vi "IQA check.vi"(8 "CHANGE":refnum<user-event>, 11 "connection in":T1) -> (3 "connection out":T1)   [LabVIEW 2017]
uses:
  <vilib>/addons/database/Connection.llb/Conn ObjectReference.ctl
  Control/State machine.ctl
  <vilib>/Utility/miscctls.llb/LVPointTypeDef.ctl
  <vilib>/addons/database/Connection.llb/Conn Execute.vi
  <vilib>/addons/database/Recordset.llb/Rec Fetch Recordset Data (R).vi
  <vilib>/addons/database/Recordset.llb/Rec Destroy - Connection.vi
  <vilib>/addons/database/_DB Variant To Data/Database Variant To Data.xnode
  <vilib>/addons/database/NI_Database_API.lvlib
  <vilib>/addons/database/Connection.llb/DB Tools Open Connec (Path).vi
panel:
  out "stock":string
  out "Ex-Im Code":string
  out "offset":string
  in  "Tab Control":enum32{"Main", "Debug"}(tab)
  in  "Level of shipment":string(combo)="N"
  in  "NG":bool
  in  "OK":bool
  out "Result":bool
  in  "Maker Code 2":string caption="Maker Code"
  out "Item Code 2":string caption="Item Code"
  in  "Barcode (F2)":string
  out "Maker Code":string
  out "Item Code":string
  in  "QR-Code (F1)":string
  out "ECODE":string
  # "IQA CHECK"
  # "QUALITY"
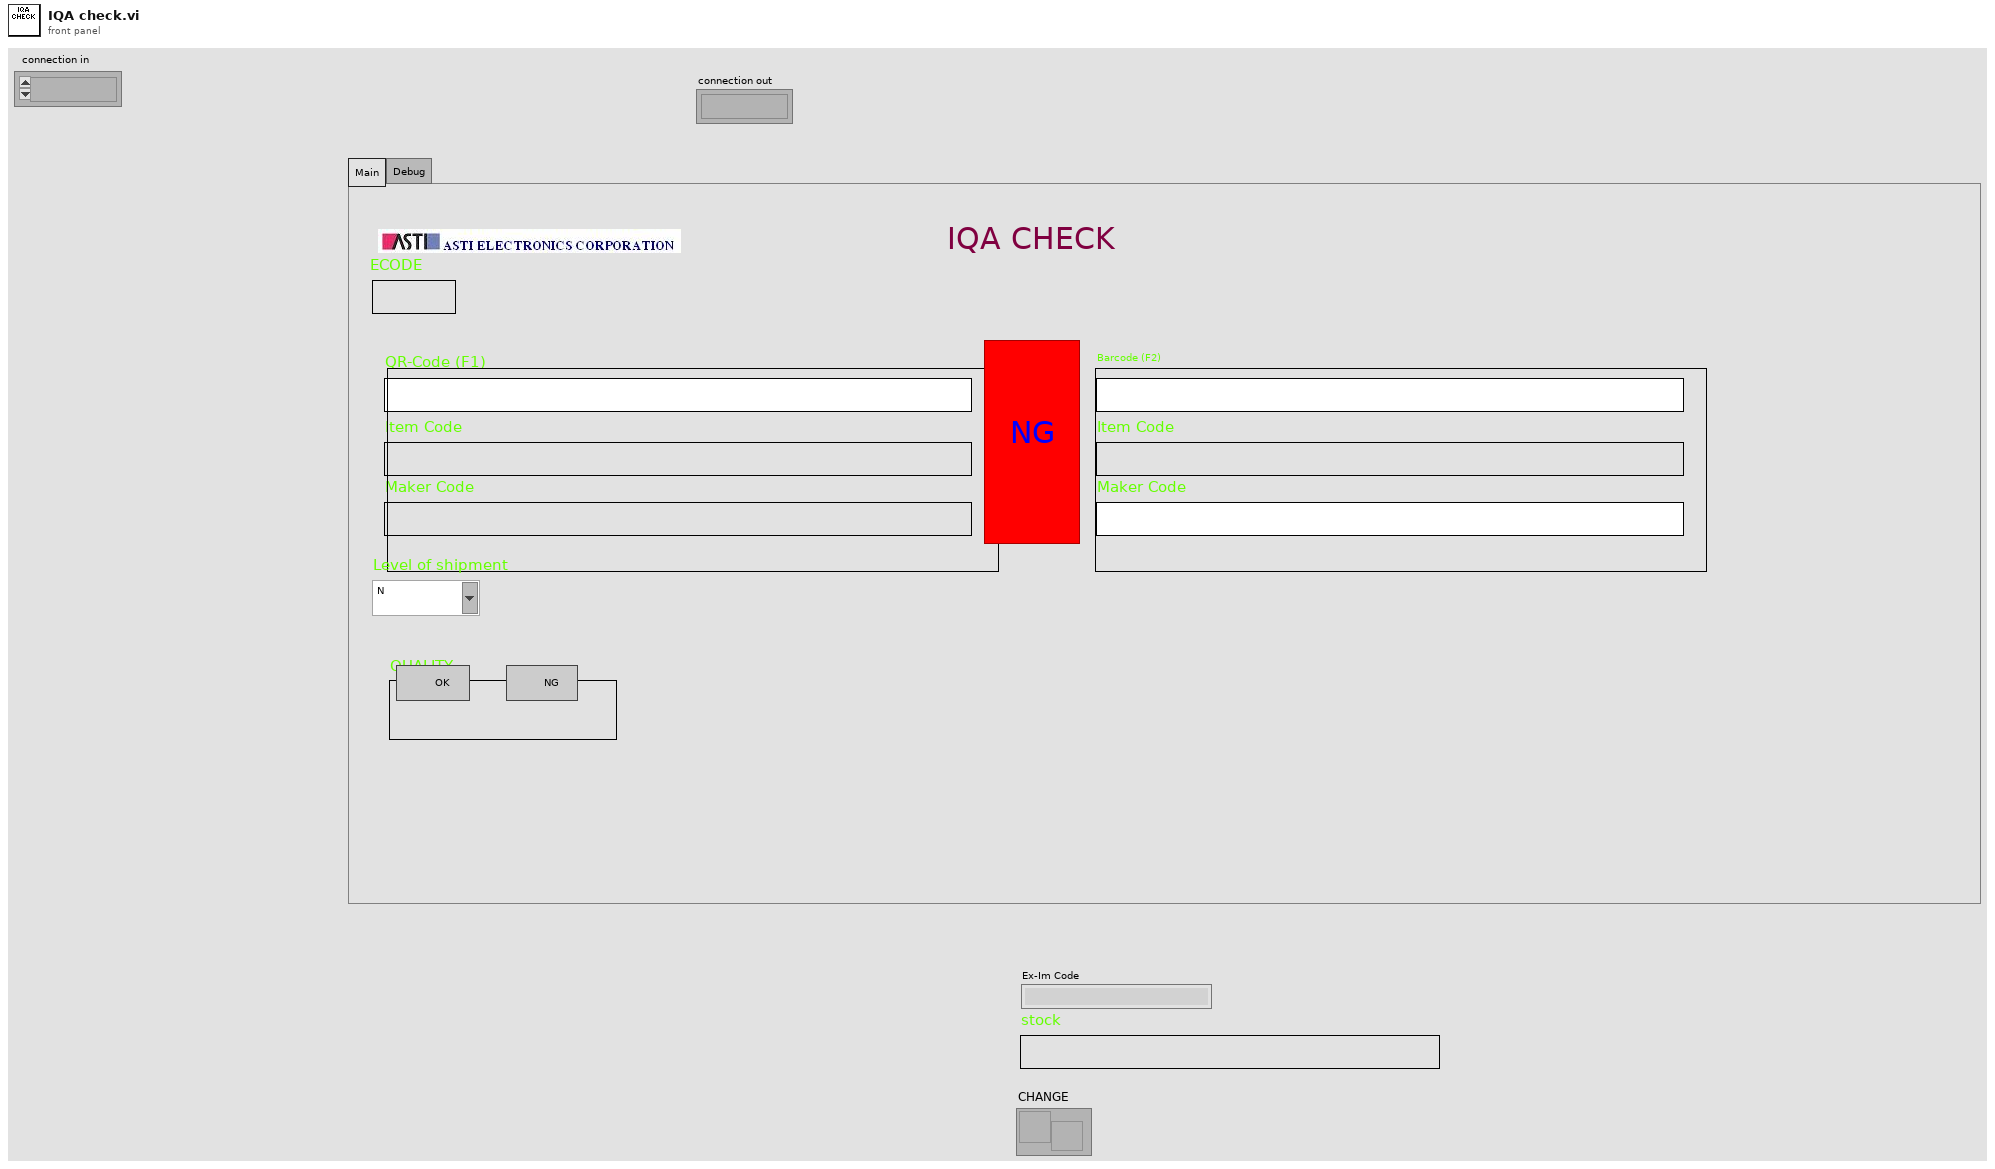
[diagram p1: front panel]
types:
  T1 = typedef "NI_Database_API.lvlib/Conn ObjectReference.ctl" = refnum<k1>
  T2 = enum8{"Enabled", "Disabled", "Disabled and Grayed Out"}
  T3 = typedef "LVPointTypeDef.ctl" = cluster{"Horizontal":i16, "Vertical":i16}
  T4 = typedef "State machine.ctl" = enum16{"Licence check", "Initial", "Log in", "Creat Config file", "Network setting", "Creat database 1", "Creat database 2", "Creat database 3", "Transfer", "Begin", "Exit"}
  T5 = typedef "NI_Database_API.lvlib/Rec ObjectReference.ctl" = refnum<k1>
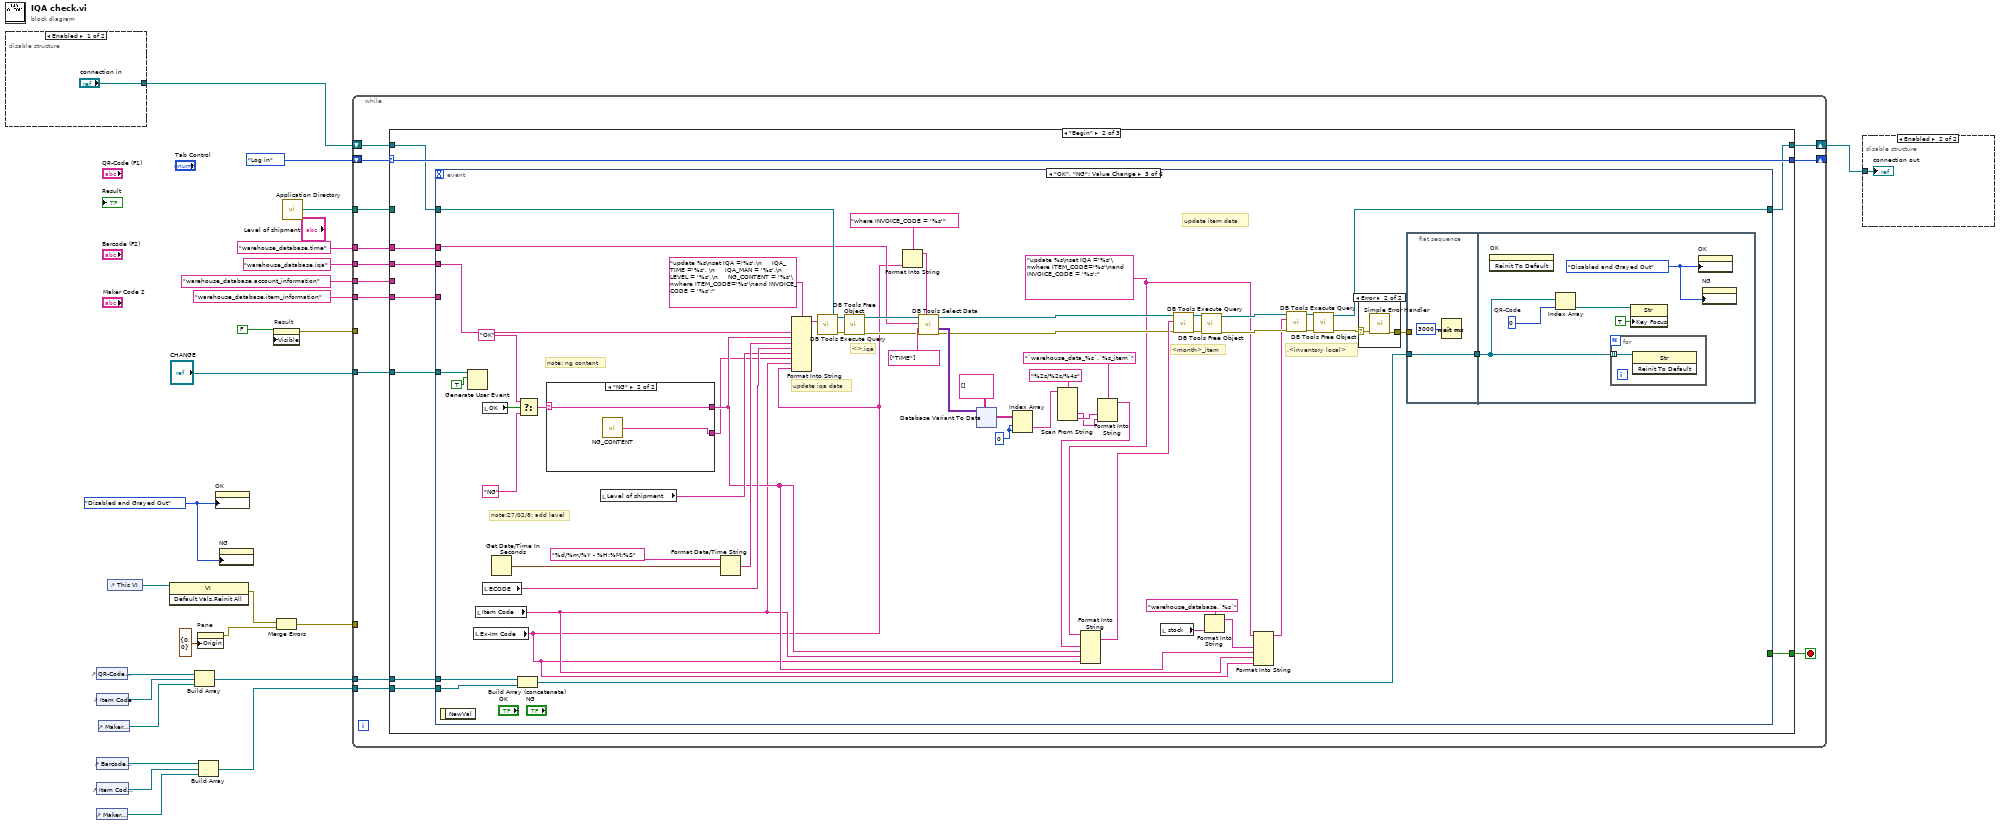
[diagram p0: block diagram]
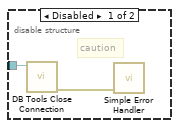
[diagram p2: hidden frame]
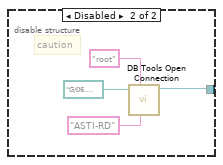
[diagram p3: hidden frame]
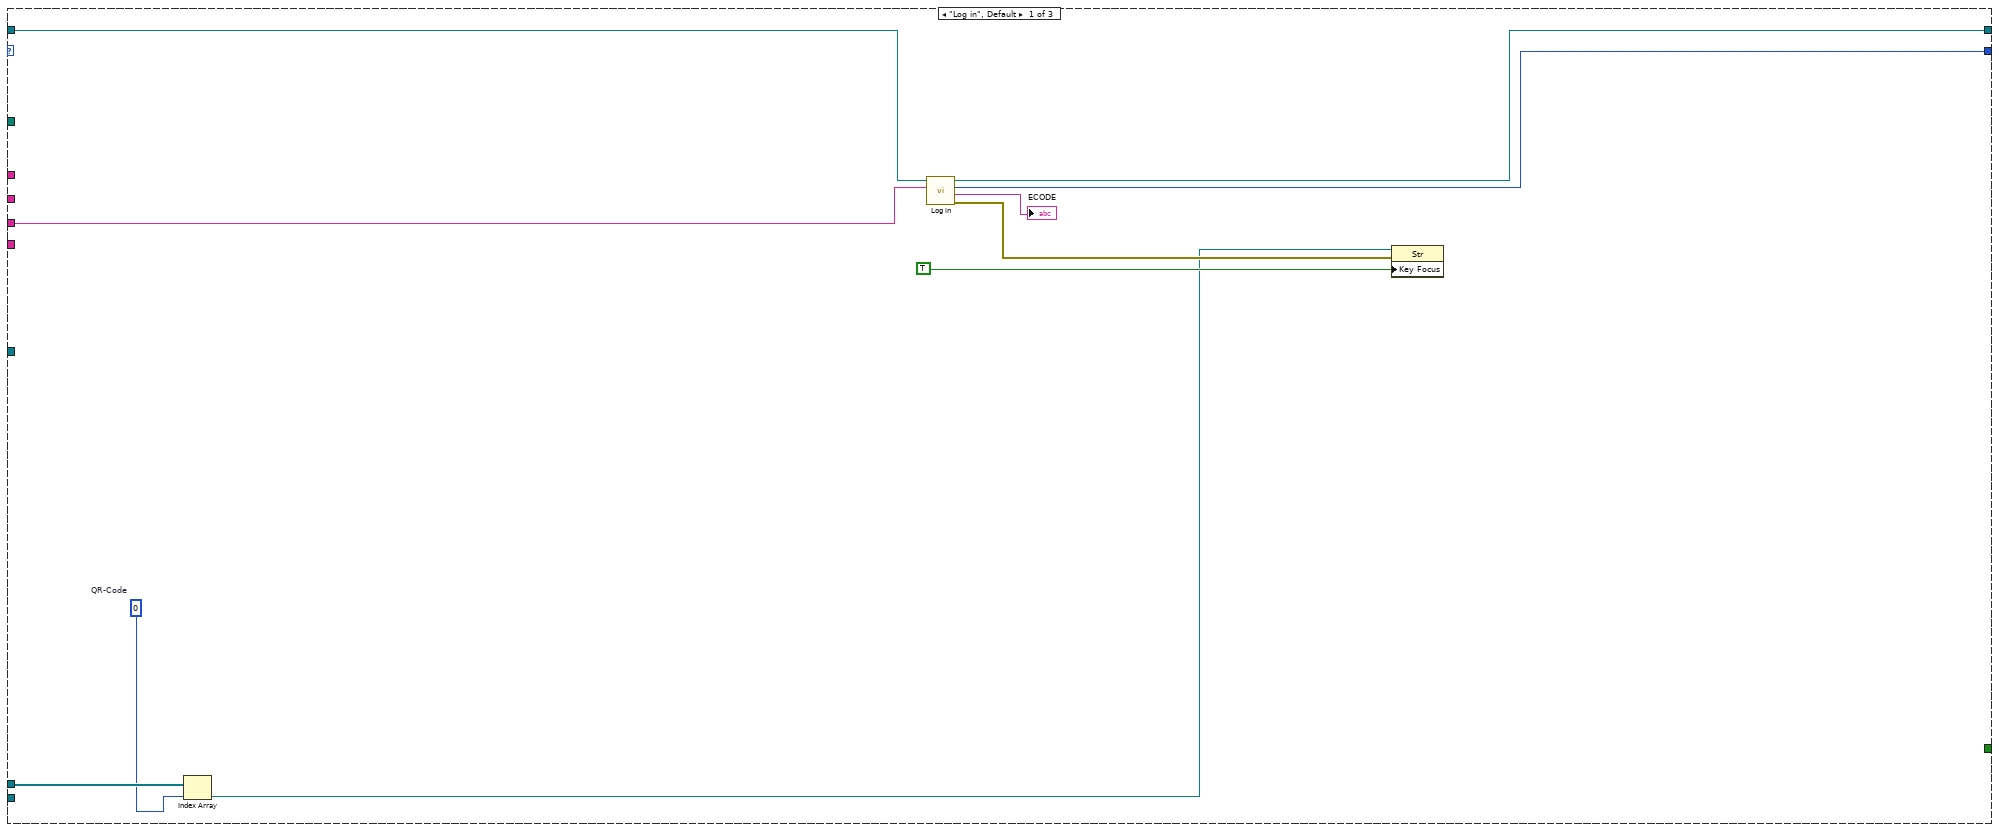
[diagram p4: hidden frame]
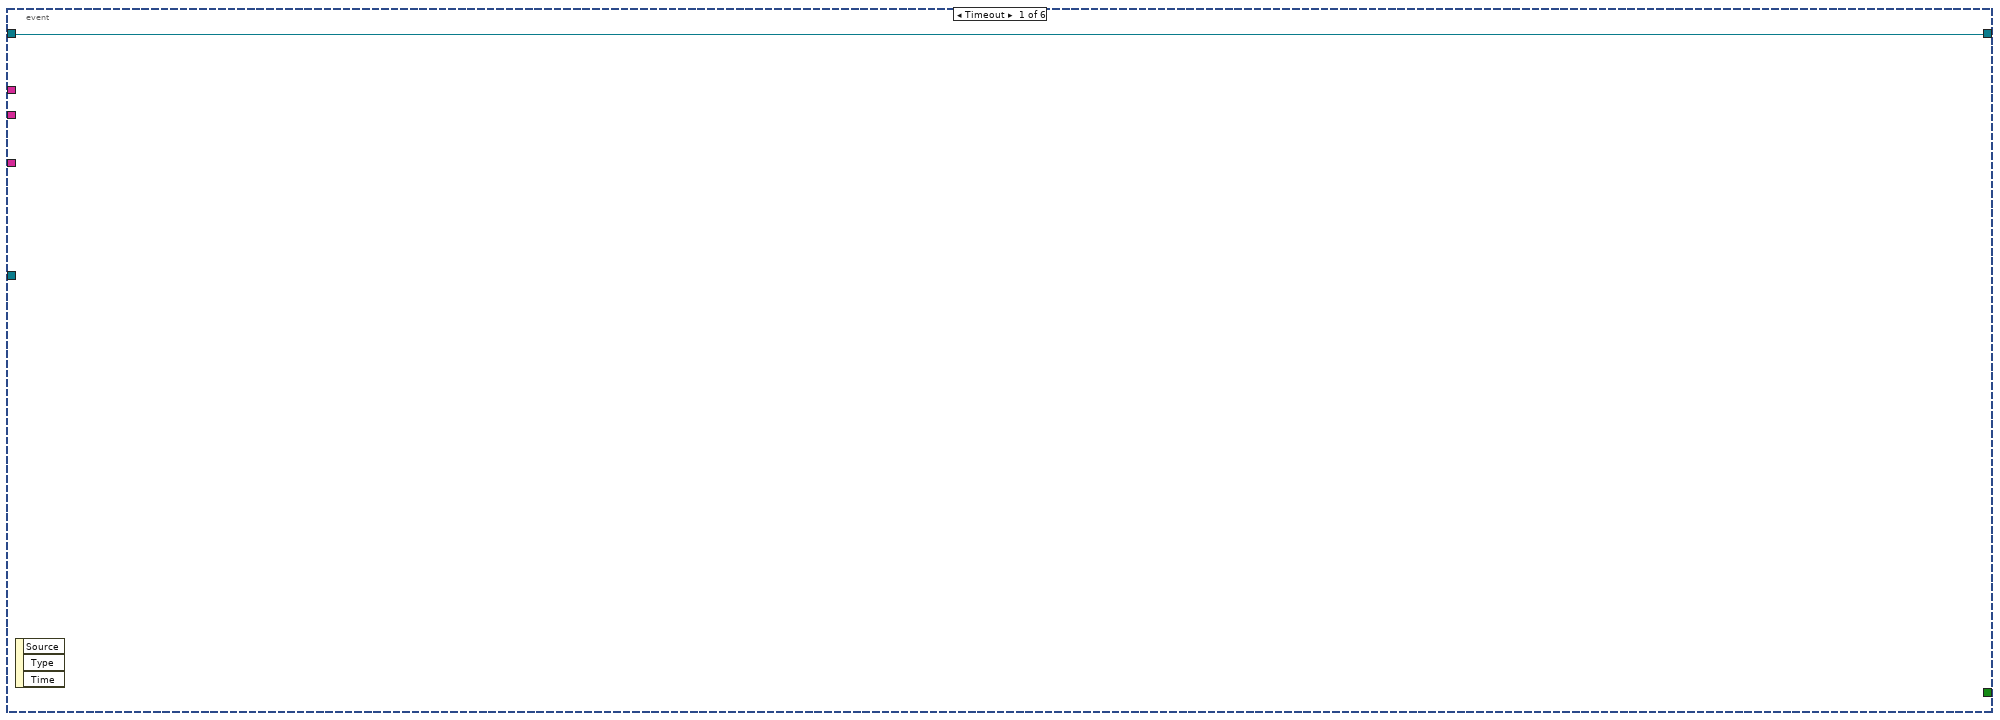
[diagram p5: hidden frame]
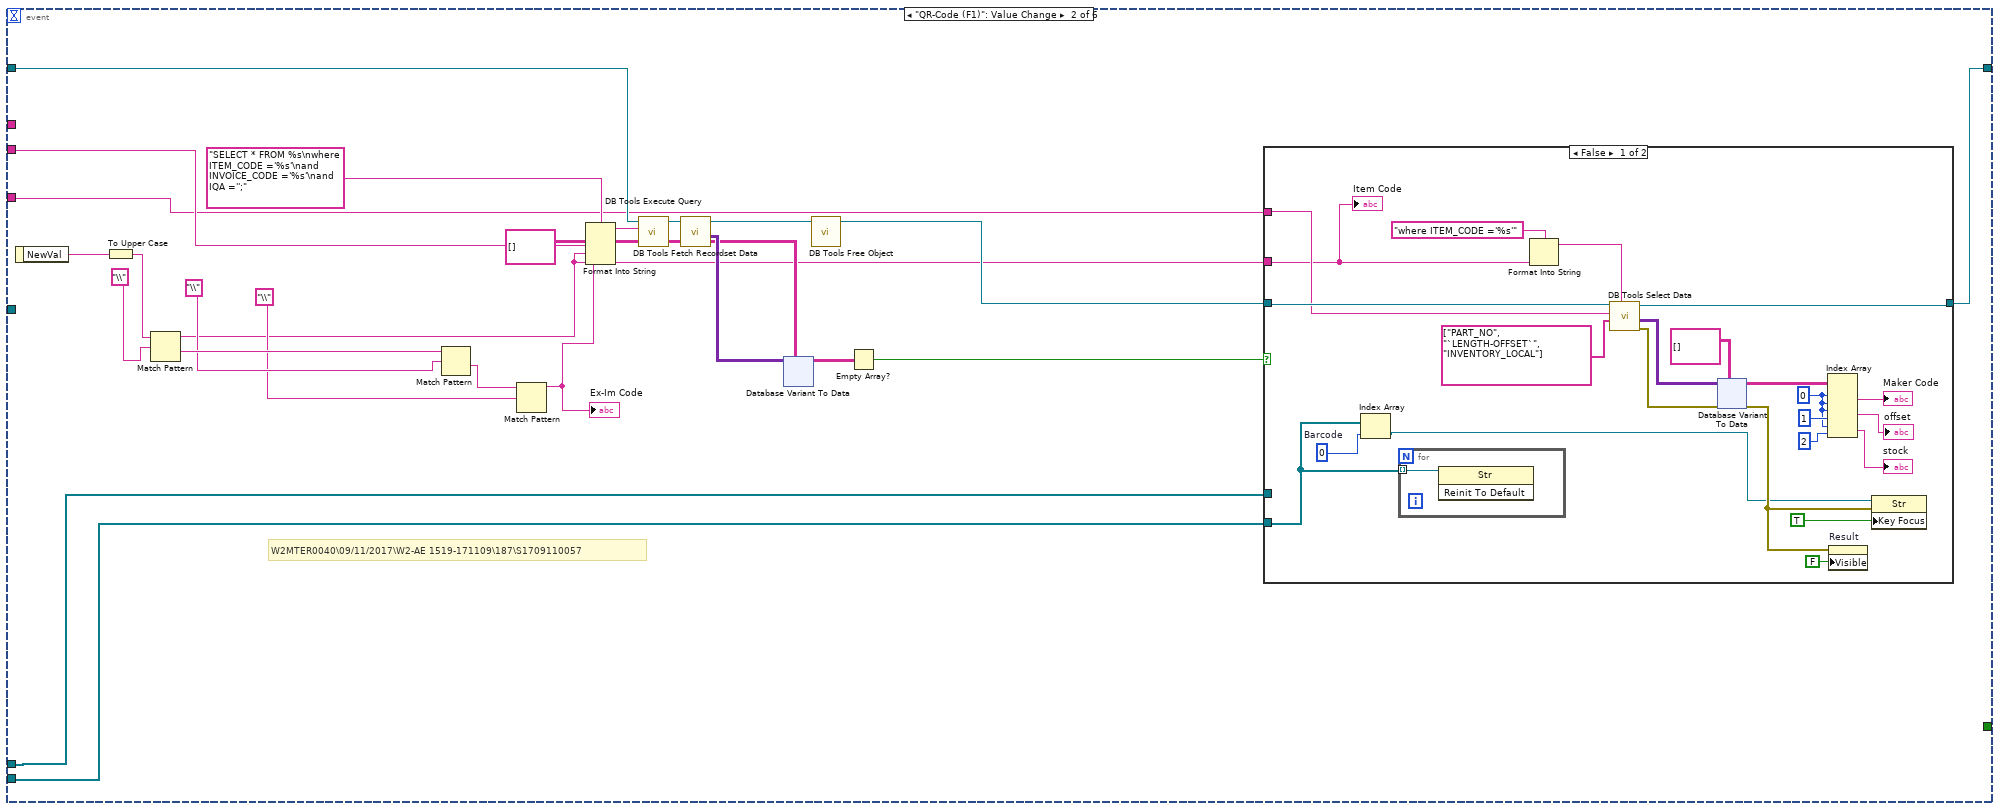
[diagram p6: hidden frame]
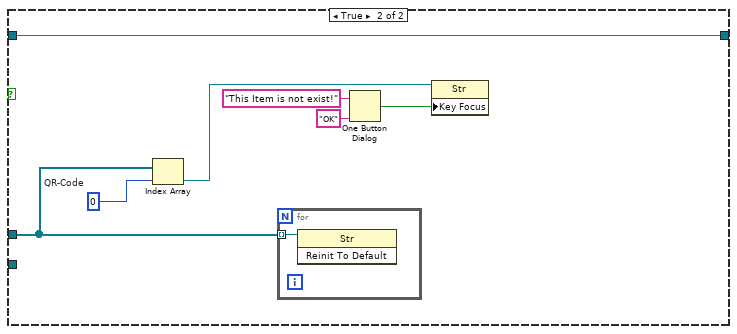
[diagram p7: hidden frame]
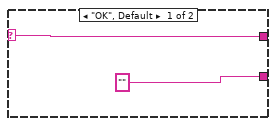
[diagram p8: hidden frame]
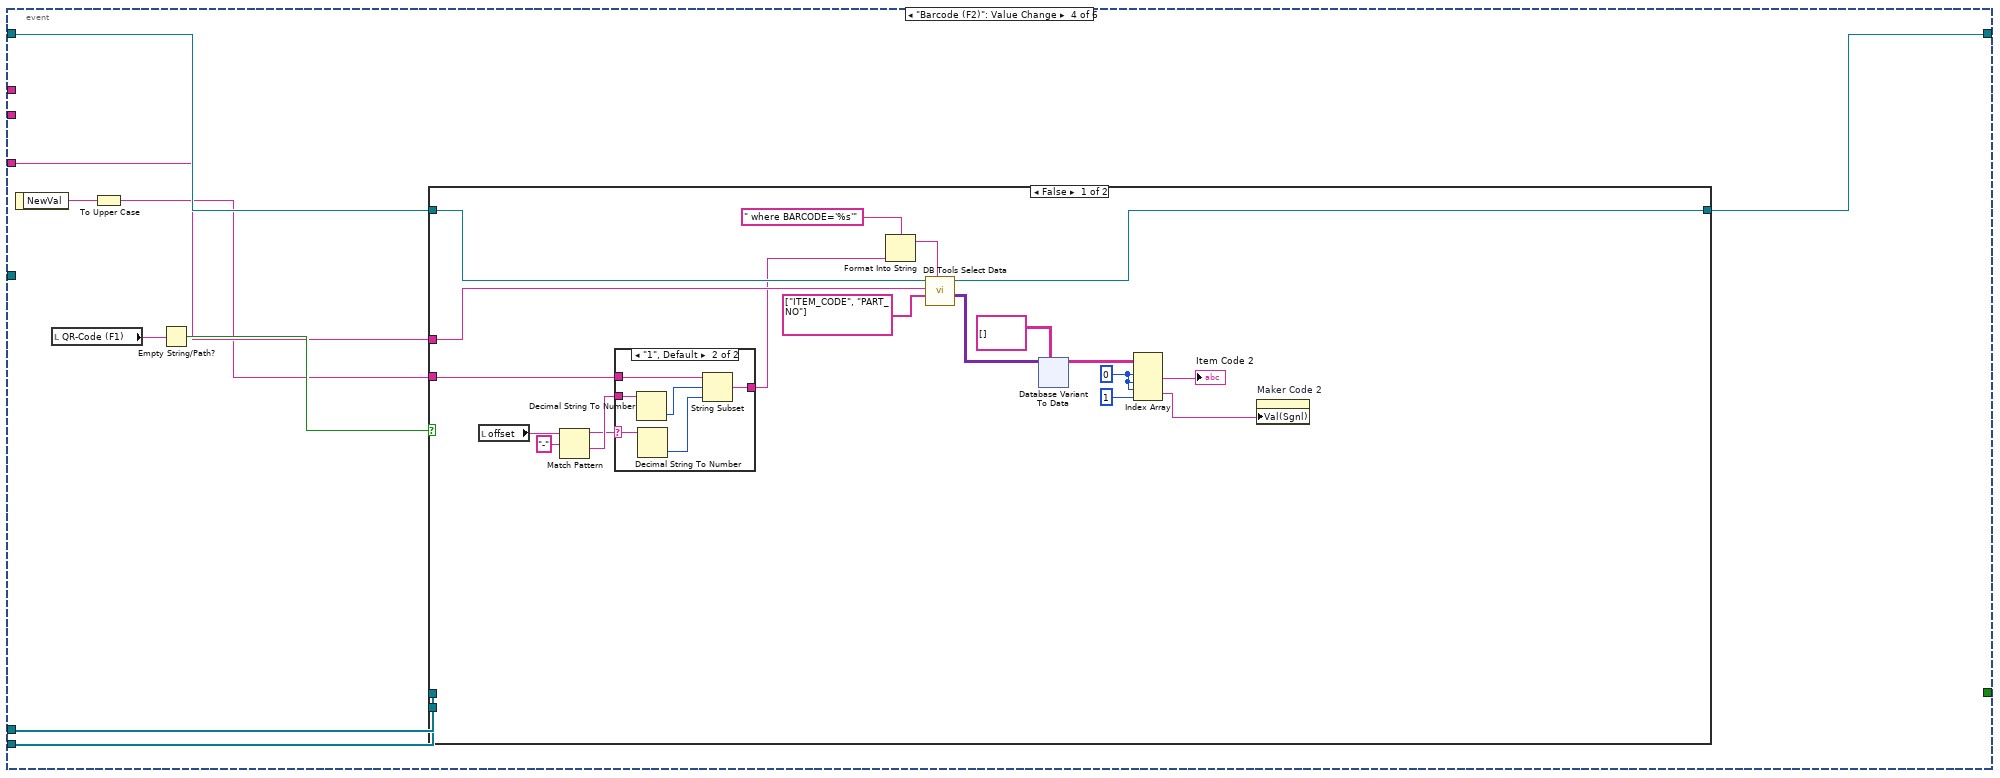
[diagram p10: hidden frame]
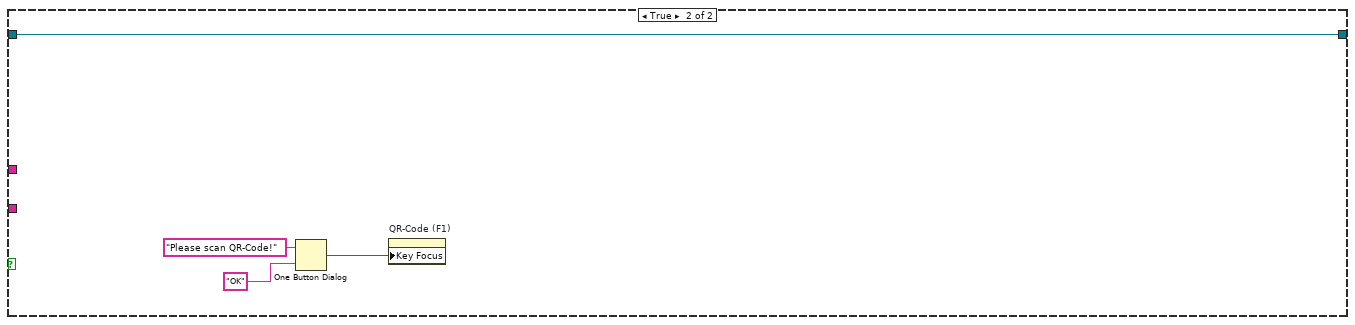
[diagram p12: hidden frame]
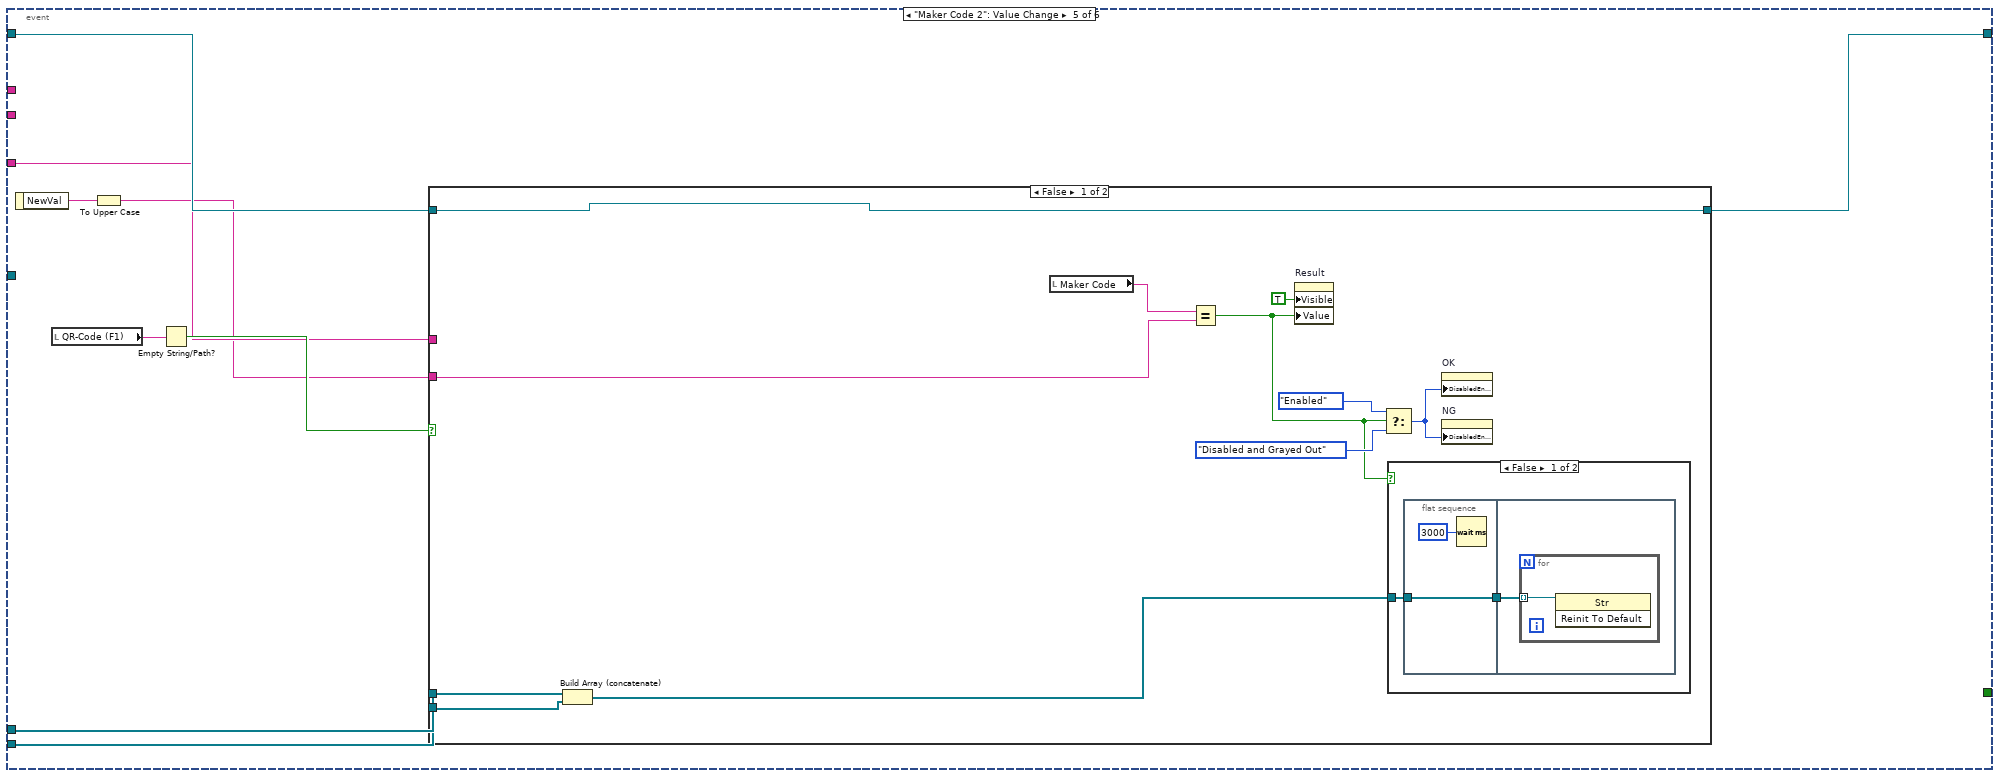
[diagram p13: hidden frame]
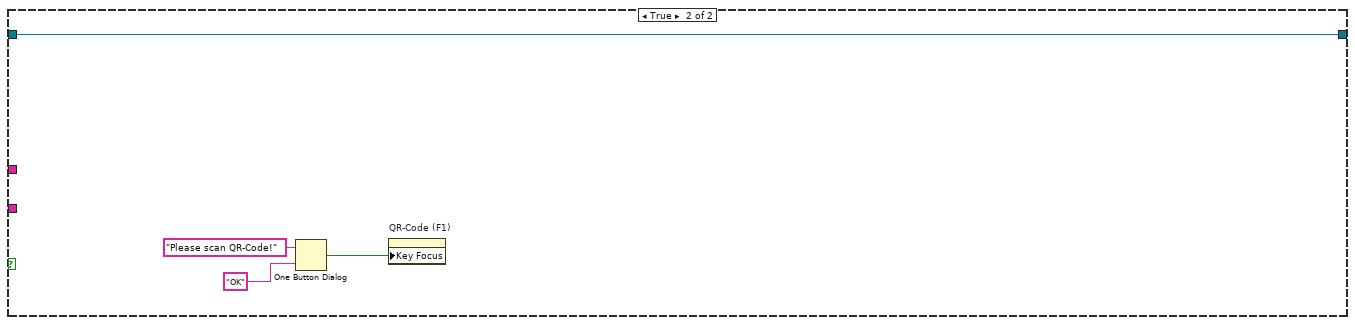
[diagram p15: hidden frame]
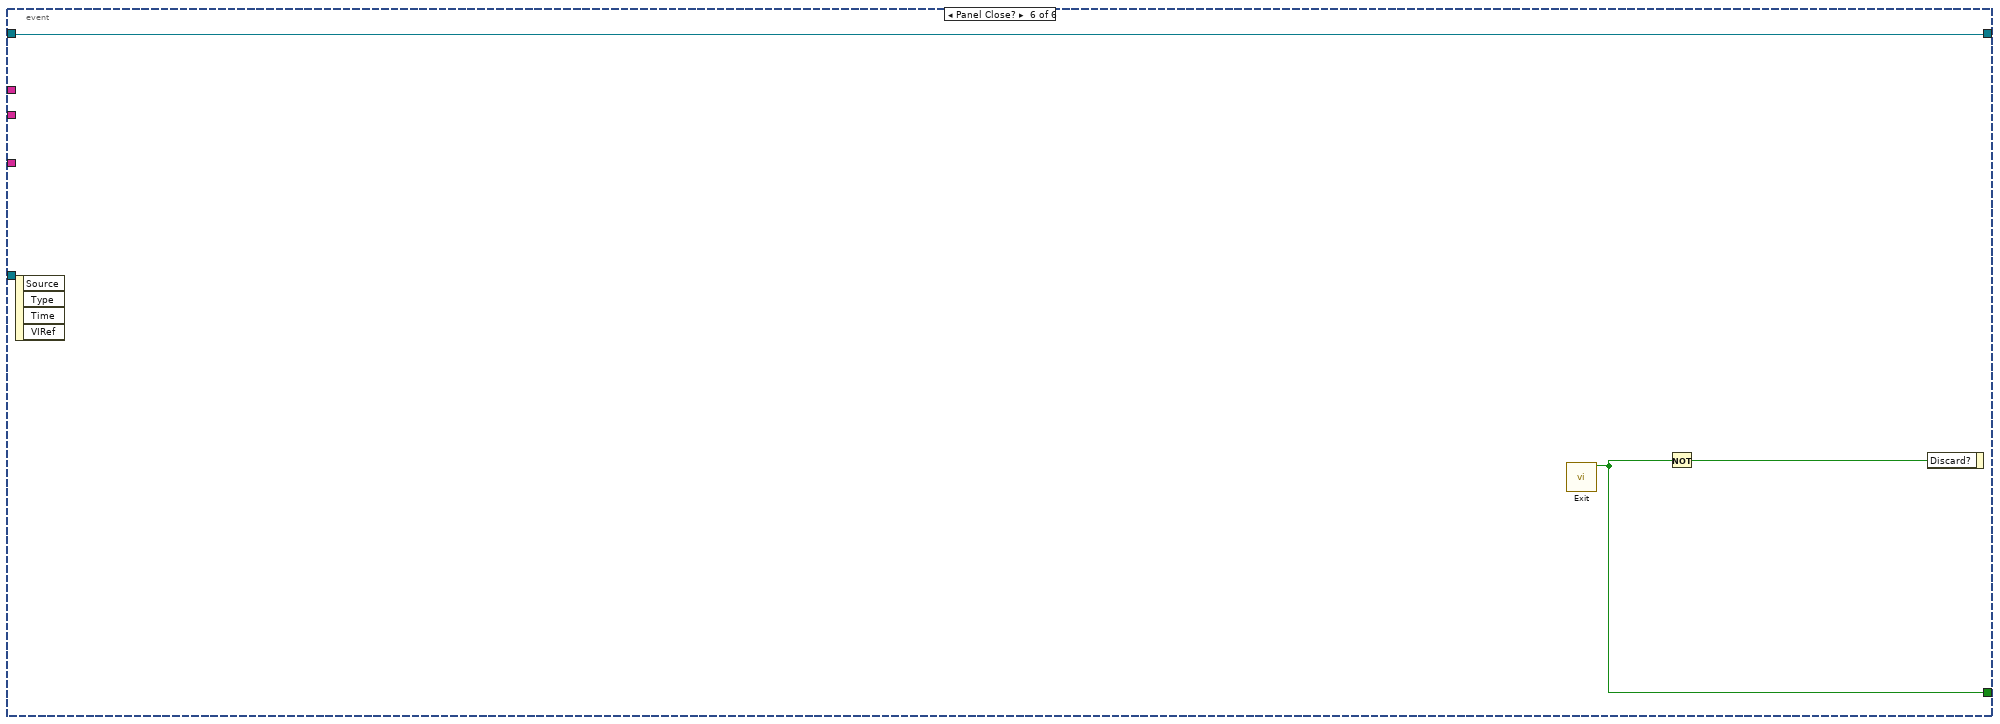
[diagram p16: hidden frame]
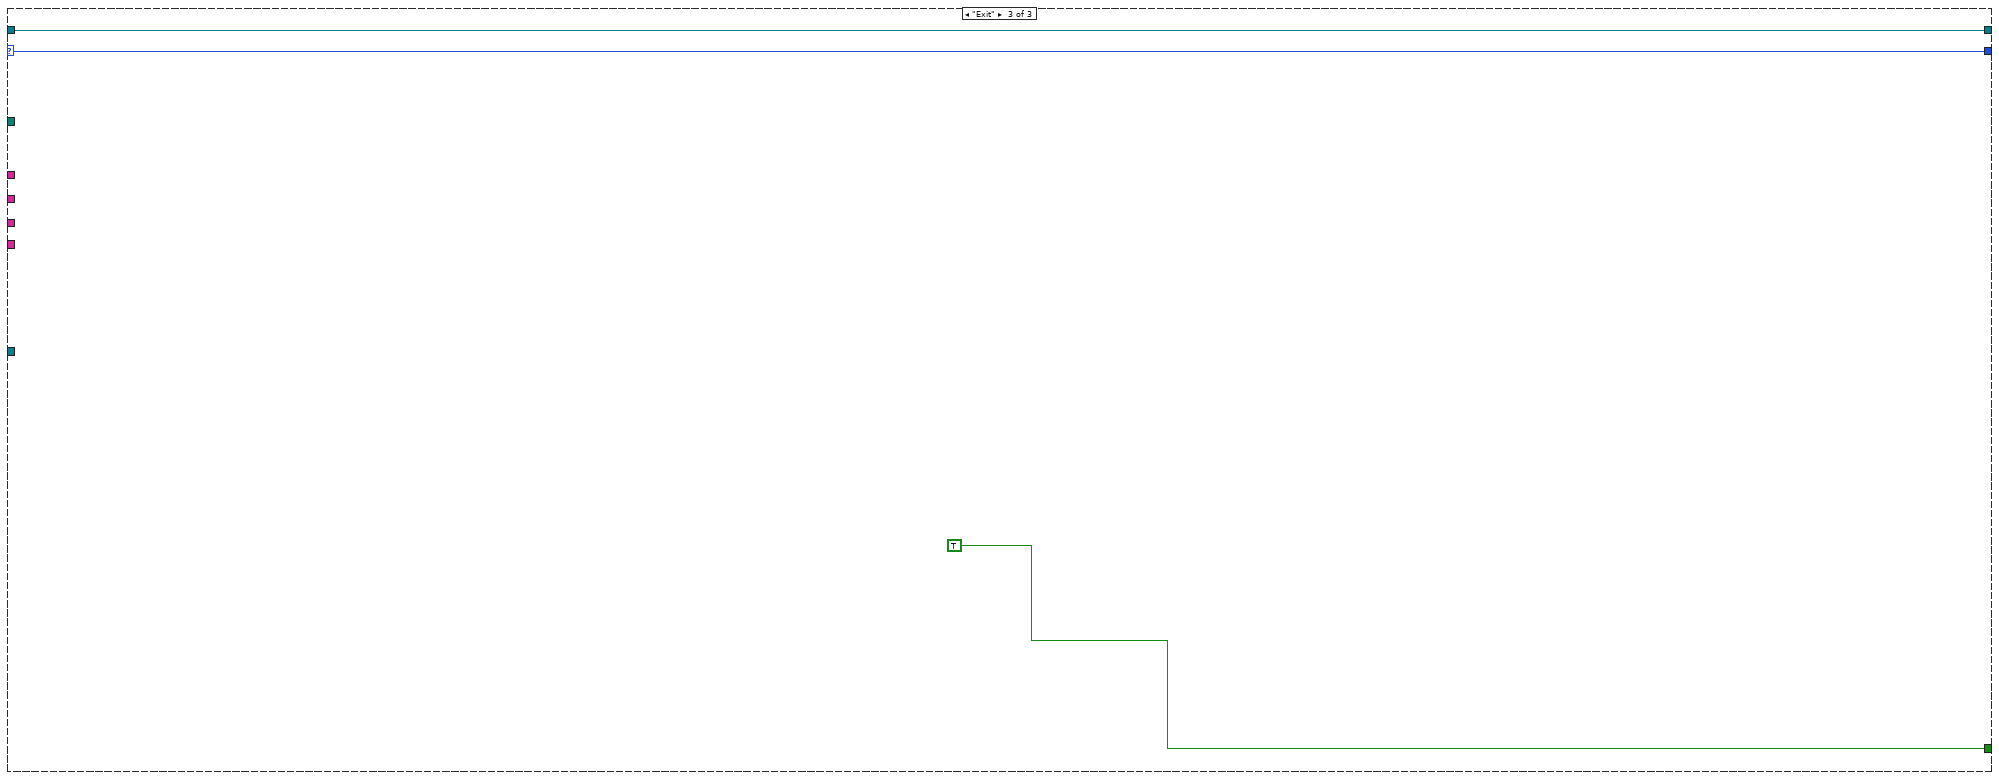
[diagram p17: hidden frame]
diagram:
  w10 = T2."Disabled and Grayed Out" ("Disabled")
  n1 = disable-structure shown="Enabled" {
    disable-tunnel: ["connection in" w30] -> w15
    frame Enabled {
    }
    frame Disabled {
      # "caution"
      n2 = call-poly <vilib>:"DB Tools Open Connection.vi"("password"="ASTI-RD", "userID"="root", "connection information"=path "G:/06. Data/Data/05. AEC/07. New Storage Management/Setting/Database local.dsn") -> ("connection reference"=w30:T1)  [unwired: 5 in, 1 out]
    }
  }
  n3 = control-ref of="QR-Code (F1)"() -> (w9:refnum<vi>)
  n4 = control-ref of="Maker Code 2"() -> (w3:refnum<vi>)
  n5 = control-ref of="Item Code"() -> (w8:refnum<vi>)
  n6 = control-ref of="Barcode (F2)"() -> (w5:refnum<vi>)
  n7 = control-ref of="Item Code 2"() -> (w4:refnum<vi>)
  n8 = control-ref of="Maker Code"() -> (w7:refnum<vi>)
  n9 = control-ref of="This VI"() -> (w22:refnum<vi>)
  n10 = invoke class="VI" method="Default Vals.Reinit All"(reference=w22) -> (error out=w20:errorcluster)  [unwired: 2 in, 2 out]
  n11 = Build Array(w9, w8, w7) -> (w6:refnum<vi>[])
  n12 = property on="Pane" class="Pane"("Origin"=T3 {"Horizontal"=0, "Vertical"=0}) -> (error out=w19:errorcluster)  [unwired: 2 in, 1 out]
  n13 = Build Array(w5, w4, w3) -> (w2:refnum<vi>[])
  n14 = property on="OK" class="Bool (strict)"("DisabledEnum"=w10) -> ()  [unwired: 2 in, 2 out]
  n15 = property on="NG" class="Bool"("DisabledEnum"=w10) -> ()  [unwired: 2 in, 2 out]
  n16 = property on="Result" class="Bool (strict)"("Visible"=FALSE) -> (error out=w11:errorcluster)  [unwired: 2 in, 1 out]
  n17 = Merge Errors(w20, w19) -> (w18:errorcluster)
  n18 = call <vilib>:"Application Directory.vi"() -> ("Application Directory"=w24:path)
  n19 = while {
    shift-right: [w40] -> _
    shift-left: State_machine."Log in" ("Enum") -> [w42]
    tunnel: w24 -> [w41]
    shift-right: [w39] -> w23
    shift-left: w15 -> [w38]
    tunnel: w18 -> [_]
    tunnel: "warehouse_database.time" ("table") -> [w37]
    tunnel: "warehouse_database.iqa" ("table") -> [w36]
    tunnel: "warehouse_database.account_information" ("table") -> [w35]
    tunnel: "warehouse_database.item_information" ("table") -> [w34]
    tunnel: w11 -> [_]
    tunnel: w6 -> [w33]
    tunnel: w2 -> [w32]
    tunnel: "CHANGE" -> [w31]
    stop <- w43 stop-if-true
    n20 = case shown="\"Begin\"" w42 {
      selector: w42 -> [_ w63 w441]
      tunnel: [_ w58 TRUE ("T button?")] -> w43
      tunnel: w41 -> [_ _ _]
      tunnel: [w50 w63 w441] -> w40
      tunnel: [w51 w60 w442] -> w39
      tunnel: w38 -> [w53 w61 w442]
      tunnel: w37 -> [_ w55 _]
      tunnel: w36 -> [_ w62 _]
      tunnel: w35 -> [w52 _ _]
      tunnel: w34 -> [_ w59 _]
      tunnel: w33 -> [w46 w57 _]
      tunnel: w32 -> [_ w56 _]
      tunnel: w31 -> [_ w54 _]
      frame "Log in", Default {
        w45 = 0  # QR-Code
        n21 = Index Array(array=w46, index=w45) -> (element=w44:refnum<vi>)
        n22 = call "Log in.vi"("String in"=w52, "Refnum in"=w53) -> ("error out"=w48:errorcluster, "String out"=→"ECODE":string, "Enum"=w50:T4, "Refnum out"=w51:T1)  [unwired: 5 in, 1 out]
        n23 = property class="Str"(reference=w44, error in=w48, "Key Focus"=TRUE) -> ()  [unwired: 2 out]
      }
      frame "Begin" {
        n24 = event shown="[2] \"OK\", \"NG\": Value Change" {
          selector: _ -> [_ _ _ _ _ _]
          dyn-events: _ -> [_ _ _ _ _ _]
          timeout: _ -> [_ _ _ _ _ _]
          tunnel: w62 -> [_ w81 w265 _ _ _]
          tunnel: w61 -> [w64 w78 w213 w330 w413 w438]
          tunnel: [w64 w70 w224 w328 w411 w438] -> w60
          tunnel: w59 -> [_ w69 _ w329 w412 _]
          tunnel: [_ _ _ _ _ w440] -> w58
          tunnel: w57 -> [_ w66 w253 w326 w409 _]
          tunnel: w56 -> [_ w65 w252 w325 w408 _]
          tunnel: w55 -> [_ _ w210 _ _ _]
          tunnel: w54 -> [_ _ w212 _ _ _]
          event Timeout {
            n25 = event-data() -> ()  [unwired: 1 in, 3 out]
          }
          event "QR-Code (F1)": Value Change {
            # "W2MTER0040\\09/11/2017\\W2-AE 1519-171109\\187\\S1709110057"
            n26 = event-data() -> ("NewVal"=w88:string)  [unwired: 1 in]
            n27 = To Upper Case(1:w88) -> (0:w67:string)
            n28 = Match Pattern(string=w67, regular expression="\\") -> (before substring=w68:string, after substring=w86:string)  [unwired: 1 in, 2 out]
            n29 = Match Pattern(string=w86, regular expression="\\") -> (after substring=w84:string)  [unwired: 1 in, 3 out]
            n30 = Match Pattern(string=w84, regular expression="\\") -> (before substring=w80:string)  [unwired: 1 in, 3 out]
            "Ex-Im Code" <- w80
            n31 = Format Into String(format string="SELECT * FROM %s\nwhere ITEM_CODE ='%s'\nand INVOICE_CODE ='%s'\nand IQA ='';", w81, w68, w80) -> (resulting string=w79:string)  [unwired: 2 in, 1 out]
            n32 = call-poly <vilib>:"DB Tools Execute Query.vi"("SQL query"=w79, "connection reference"=w78) -> ("recordset reference"=w77:T5)  [unwired: 6 in, 1 out]
            n33 = call-poly <vilib>:"DB Tools Fetch Recordset Data.vi"("recordset reference"=w77) -> ("recordset data"=w75:variant[][], "recordset reference out"=w76:T5)  [unwired: 4 in, 1 out]
            n34 = xnode "Database Variant To Data"("database variant"=w75, "type"=string[][] []) -> ("data"=w73:string[][])  [unwired: 1 in, 1 out]
            n35 = call-poly <vilib>:"DB Tools Free Object.vi"("recordset reference"=w76) -> ("connection reference"=w71:T1)  [unwired: 9 in, 1 out]
            n36 = Empty Array?(array=w73) -> (empty?=w72:bool)
            n37 = case shown="False" w72 {
              tunnel: w71 -> [w111 w161]
              tunnel: [w109 w161] -> w70
              tunnel: w69 -> [w110 _]
              tunnel: w68 -> [w105 _]
              tunnel: w66 -> [_ w159]
              tunnel: w65 -> [w94 _]
              frame False {
                w93 = 0  # Barcode
                w91 = 0 ("index (row)")
                n38 = Index Array(array=w94, index=w93) -> (element=w92:refnum<vi>)
                n39 = for {
                  tunnel: w94 -> [w112] mode=indexing
                  n40 = invoke class="Str" method="Reinit To Default"(reference=w112) -> ()  [unwired: 2 in, 3 out]
                }
                n41 = Format Into String(format string="where ITEM_CODE ='%s'", w105) -> (resulting string=w106:string)  [unwired: 2 in, 1 out]
                n42 = call <vilib>:"DB Tools Select Data.vi"("condition"=w106, "columns"=string[] ["PART_NO", "`LENGTH-OFFSET`", "INVENTORY_LOCAL"], "table"=w110, "connection reference"=w111) -> ("error out"=w98:errorcluster, "data"=w104:variant[][], "connection reference out"=w109:T1)  [unwired: 2 in]
                n43 = xnode "Database Variant To Data"("database variant"=w104, "error in (no error)"=w98, "type"=string[][] []) -> ("data"=w102:string[][], "error out"=w96:errorcluster)
                n44 = Index Array(array=w102, index (row) #1=w91, index (col) #1=w91, index (row) #2=w91, index (col) #2=1 ("disabled index (col)"), index (row) #3=w91, index (col) #3=2 ("disabled index (col)")) -> (element #1=→"Maker Code":string, element #2=→"offset":string, element #3=→"stock":string)
                n45 = property on="Result" class="Bool (strict)"(error in=w96, "Visible"=FALSE) -> ()  [unwired: 1 in, 2 out]
                n46 = property class="Str"(reference=w92, error in=w96, "Key Focus"=TRUE) -> ()  [unwired: 2 out]
                "Item Code" <- w105
              }
              frame True {
                w158 = 0  # QR-Code
                n47 = Index Array(array=w159, index=w158) -> (element=w157:refnum<vi>)
                n48 = for {
                  tunnel: w159 -> [w164] mode=indexing
                  n49 = invoke class="Str" method="Reinit To Default"(reference=w164) -> ()  [unwired: 2 in, 3 out]
                }
                n50 = One Button Dialog(message="This Item is not exist!", button name ("OK")="OK") -> (true=w160:bool)
                n51 = property class="Str"(reference=w157, "Key Focus"=w160) -> ()  [unwired: 1 in, 2 out]
              }
            }
          }
          event "OK", "NG": Value Change {
            w239 = 0 ("index (row)")
            w223 = "update %s\nset IQA ='%s'\nwhere ITEM_CODE='%s'\nand INVOICE_CODE = '%s';"
            # "note: ng content"
            # "<month>_item"
            # "<>.iqa"
            # "note:27/02/8: add level"
            # ".<inventory local>"
            # "update item data"
            # "update iqa data"
            n52 = event-data() -> ()  [unwired: 1 in, 1 out]
            n53 = Generate User Event(user event=w212, event data cluster=TRUE ("event data")) -> ()  [unwired: 2 in, 2 out]
            n54 = local read "Ex-Im Code"() -> (w209:string)
            n55 = local read "Item Code"() -> (w215:string)
            n56 = local read "OK"() -> (w264:bool)
            n57 = local read "ECODE"() -> (w258:string)
            n58 = Get Date/Time In Seconds() -> (seconds since 1Jan1904=w261:timestamp)
            n59 = Build Array (concatenate)(w253, w252) -> (w250:refnum<vi>[])
            n60 = Select(t="OK", s=w264, f="NG") -> (s? t:f=w217:string)
            n61 = case shown="\"NG\"" w217 {
              selector: w217 -> [w268 w270]
              tunnel: [w268 w270] -> w216
              tunnel: ["" w269] -> w214
              frame "OK", Default {
              }
              frame "NG" {
                n62 = call "NG_CONTENT.vi"() -> ("STR 2"=w269:string)  [unwired: 1 in]
              }
            }
            n63 = local read "Level of shipment"() -> (w218:string)
            n64 = Format Date/Time String(time format string (%c)="%d/%m/%Y - %H:%M:%S", seconds (now)=w261) -> (date/time string=w259:string)  [unwired: 1 in]
            n65 = Format Into String(format string="update %s\nset IQA ='%s',\n     IQA_TIME ='%s', \n     IQA_MAN = '%s',\n     LEVEL = '%s',\n     NG_CONTENT = '%s'\nwhere ITEM_CODE='%s'\nand INVOICE_CODE = '%s';", w265, w216, w259, w258, w218, w214, w215, w209) -> (resulting string=w257:string)  [unwired: 2 in, 1 out]
            n66 = call-poly <vilib>:"DB Tools Execute Query.vi"("SQL query"=w257, "connection reference"=w213) -> ("error out"=w255:errorcluster, "recordset reference"=w256:T5)  [unwired: 6 in]
            n67 = call-poly <vilib>:"DB Tools Free Object.vi"("error in (no error)"=w255, "recordset reference"=w256) -> ("error out"=w231:errorcluster, "connection reference"=w243:T1)  [unwired: 8 in]
            n68 = Format Into String(format string="where INVOICE_CODE = '%s'", w209) -> (resulting string=w244:string)  [unwired: 2 in, 1 out]
            n69 = call <vilib>:"DB Tools Select Data.vi"("condition"=w244, "error in (no error)"=w231, "columns"=string[] ["TIME"], "table"=w210, "connection reference"=w243) -> ("error out"=w230:errorcluster, "data"=w242:variant[][], "connection reference out"=w234:T1)  [unwired: 1 in]
            n70 = xnode "Database Variant To Data"("database variant"=w242, "type"=string[][] []) -> ("data"=w240:string[][])  [unwired: 1 in, 1 out]
            n71 = Index Array(array=w240, index (row)=w239, index (col)=w239) -> (element=w238:string)
            n72 = Scan From String(format string="%2s/%2s/%4s", input string=w238) -> (output 2=w232:string, output 3=w233:string)  [unwired: 6 in, 3 out]
            n73 = Format Into String(format string="`warehouse_data_%s`.`%s_item`", w233, w232) -> (resulting string=w235:string)  [unwired: 2 in, 1 out]
            n74 = Format Into String(format string=w223, w235, w216, w215, w209) -> (resulting string=w247:string)  [unwired: 2 in, 1 out]
            n75 = local read "stock"() -> (w221:string)
            n76 = call-poly <vilib>:"DB Tools Execute Query.vi"("error in (no error)"=w230, "SQL query"=w247, "connection reference"=w234) -> ("error out"=w249:errorcluster, "recordset reference"=w248:T5)  [unwired: 5 in]
            n77 = call-poly <vilib>:"DB Tools Free Object.vi"("error in (no error)"=w249, "recordset reference"=w248) -> ("error out"=w228:errorcluster, "connection reference"=w225:T1)  [unwired: 8 in]
            n78 = Format Into String(format string="warehouse_database.`%s`" ("table"), w221) -> (resulting string=w220:string)  [unwired: 2 in, 1 out]
            n79 = Format Into String(format string=w223, w220, w216, w215, w209) -> (resulting string=w219:string)  [unwired: 2 in, 1 out]
            n80 = call-poly <vilib>:"DB Tools Execute Query.vi"("error in (no error)"=w228, "SQL query"=w219, "connection reference"=w225) -> ("error out"=w227:errorcluster, "recordset reference"=w229:T5)  [unwired: 5 in]
            n81 = call-poly <vilib>:"DB Tools Free Object.vi"("error in (no error)"=w227, "recordset reference"=w229) -> ("error out"=w226:errorcluster, "connection reference"=w224:T1)  [unwired: 8 in]
            n82 = case shown="Error" w226 {
              selector: w226 -> [_ w316]
              tunnel: [_ w315] -> w254
              frame No Error {
              }
              frame Error {
                n83 = call <vilib>:"Simple Error Handler.vi"("error in (no error)"=w316) -> ("error out"=w315:errorcluster)  [unwired: 4 in, 4 out]
              }
            }
            n84 = flat-sequence {
              tunnel: w254 -> [_]
              tunnel: [w317] -> w251
              tunnel: w250 -> [w317]
              tunnel: w251 -> [w322]
              frame #0 {
                n85 = Wait (ms)(milliseconds to wait=u32 3000) -> ()  [unwired: 1 out]
              }
              frame #1 {
                w321 = 0  # QR-Code
                w323 = T2."Disabled and Grayed Out" ("Disabled")
                n86 = invoke on="OK" class="Bool (strict)" method="Reinit To Default"() -> ()  [unwired: 3 in, 3 out]
                n87 = Index Array(array=w322, index=w321) -> (element=w320:refnum<vi>)
                n88 = for {
                  tunnel: w322 -> [w324] mode=indexing
                  n89 = invoke class="Str" method="Reinit To Default"(reference=w324) -> ()  [unwired: 2 in, 3 out]
                }
                n90 = property class="Str"(reference=w320, "Key Focus"=TRUE) -> ()  [unwired: 1 in, 2 out]
                n91 = property on="OK" class="Bool (strict)"("DisabledEnum"=w323) -> ()  [unwired: 2 in, 2 out]
                n92 = property on="NG" class="Bool"("DisabledEnum"=w323) -> ()  [unwired: 2 in, 2 out]
              }
            }
          }
          event "Barcode (F2)": Value Change {
            n93 = event-data() -> ("NewVal"=w331:string)  [unwired: 1 in]
            n94 = local read "QR-Code (F1)"() -> (w333:string)
            n95 = To Upper Case(1:w331) -> (0:w327:string)
            n96 = Empty String/Path?(string/path=w333) -> (empty?=w332:bool)
            n97 = case shown="False" w332 {
              tunnel: w327 -> [w348 _]
              tunnel: w330 -> [w347 w404]
              tunnel: w329 -> [w346 _]
              tunnel: [w336 w404] -> w328
              tunnel: w326 -> [_ _]
              tunnel: w325 -> [_ _]
              frame False {
                w338 = 0 ("index (row)")
                n98 = local read "offset"() -> (w349:string)
                n99 = Match Pattern(string=w349, regular expression="-") -> (before substring=w351:string, after substring=w352:string)  [unwired: 1 in, 2 out]
                n100 = case shown="\"1\", Default" w351 {
                  selector: w351 -> [_ w400]
                  tunnel: w348 -> [w397 w403]
                  tunnel: [w397 w402] -> w343
                  tunnel: w352 -> [_ w398]
                  frame "", "0" {
                  }
                  frame "1", Default {
                    n101 = Decimal String To Number(string=w398) -> (number=w401:i32)  [unwired: 2 in, 1 out]
                    n102 = Decimal String To Number(string=w400) -> (number=w399:i32)  [unwired: 2 in, 1 out]
                    n103 = String Subset(string=w403, offset (0)=w401, length (rest)=w399) -> (substring=w402:string)
                  }
                }
                n104 = Format Into String(format string=" where BARCODE='%s'" ("condition"), w343) -> (resulting string=w342:string)  [unwired: 2 in, 1 out]
                n105 = call <vilib>:"DB Tools Select Data.vi"("condition"=w342, "columns"=string[] ["ITEM_CODE", "PART_NO"], "table"=w346, "connection reference"=w347) -> ("data"=w341:variant[][], "connection reference out"=w336:T1)  [unwired: 2 in, 1 out]
                n106 = xnode "Database Variant To Data"("database variant"=w341, "type"=string[][] []) -> ("data"=w339:string[][])  [unwired: 1 in, 1 out]
                n107 = Index Array(array=w339, index (row) #1=w338, index (col) #1=w338, index (row) #2=w338, index (col) #2=1 ("index (row)")) -> (element #1=→"Item Code 2":string, element #2=w334:string)
                n108 = property on="Maker Code 2" class="Str"("Val(Sgnl)"=w334) -> ()  [unwired: 2 in, 2 out]
              }
              frame True {
                n109 = One Button Dialog(message="Please scan QR-Code!", button name ("OK")="OK") -> (true=w405:bool)
                n110 = property on="QR-Code (F1)" class="Str"("Key Focus"=w405) -> ()  [unwired: 2 in, 2 out]
              }
            }
          }
          event "Maker Code 2": Value Change {
            n111 = event-data() -> ("NewVal"=w414:string)  [unwired: 1 in]
            n112 = local read "QR-Code (F1)"() -> (w416:string)
            n113 = To Upper Case(1:w414) -> (0:w410:string)
            n114 = Empty String/Path?(string/path=w416) -> (empty?=w415:bool)
            n115 = case shown="False" w415 {
              tunnel: w410 -> [w417 _]
              tunnel: w413 -> [w427 w434]
              tunnel: w412 -> [_ _]
              tunnel: [w427 w434] -> w411
              tunnel: w409 -> [w420 _]
              tunnel: w408 -> [w419 _]
              frame False {
                n116 = Build Array (concatenate)(w420, w419) -> (w418:refnum<vi>[])
                n117 = local read "Maker Code"() -> (w426:string)
                n118 = Equal?(x=w426, y=w417) -> (x = y?=w421:bool)
                n119 = property on="Result" class="Bool (strict)"("Visible"=TRUE, "Value"=w421) -> ()  [unwired: 2 in, 2 out]
                n120 = Select(t=T2."Enabled", s=w421, f=T2."Disabled and Grayed Out" ("Disabled")) -> (s? t:f=w424:T2)
                n121 = case shown="False" w421 {
                  tunnel: w418 -> [w429 _]
                  frame False {
                    n122 = flat-sequence {
                      tunnel: w429 -> [w430]
                      tunnel: [w430] -> w428
                      tunnel: w428 -> [w432]
                      frame #0 {
                        n123 = Wait (ms)(milliseconds to wait=u32 3000) -> ()  [unwired: 1 out]
                      }
                      frame #1 {
                        n124 = for {
                          tunnel: w432 -> [w433] mode=indexing
                          n125 = invoke class="Str" method="Reinit To Default"(reference=w433) -> ()  [unwired: 2 in, 3 out]
                        }
                      }
                    }
                  }
                  frame True {
                  }
                }
                n126 = property on="OK" class="Bool (strict)"("DisabledEnum"=w424) -> ()  [unwired: 2 in, 2 out]
                n127 = property on="NG" class="Bool"("DisabledEnum"=w424) -> ()  [unwired: 2 in, 2 out]
              }
              frame True {
                n128 = One Button Dialog(message="Please scan QR-Code!", button name ("OK")="OK") -> (true=w435:bool)
                n129 = property on="QR-Code (F1)" class="Str"("Key Focus"=w435) -> ()  [unwired: 2 in, 2 out]
              }
            }
          }
          event Panel Close? {
            n130 = event-data() -> ()  [unwired: 1 in, 4 out]
            n131 = call "Exit.vi"() -> ("T button?"=w440:bool)  [unwired: 11 in]
            n132 = Not(x=w440) -> (.not. x?=w439:bool)
            n133 = event-data("Discard?"=w439) -> ()  [unwired: 1 in, 1 out]
          }
        }
      }
      frame "Exit" {
      }
    }
  }
  n134 = disable-structure shown="Enabled" {
    disable-tunnel: w23 -> [w445 w446]
    frame Disabled {
      # "caution"
      n135 = call <vilib>:"DB Tools Close Connection.vi"("connection reference"=w445) -> ("error out"=w444:errorcluster)  [unwired: 6 in]
      n136 = call <vilib>:"Simple Error Handler.vi"("error in (no error)"=w444) -> ()  [unwired: 4 in, 5 out]
    }
    frame Enabled {
      "connection out" <- w446
    }
  }
